vi "ZSlice compute-core.vi"(6 "ZStage Pos":dbl, 7 "Objective Pos Locked":bool, 8 "error in (no error)":errorcluster, 9 "ZStep":dbl, 10 "ZStop":dbl, 11 "ZStart":dbl) -> (0 "error out":errorcluster, 1 "Motor Z Planes(um)":dbl[](array[numeric]) format="%#_12f", 2 "# of Z-planes":i32, 3 "AOL Z Planes(um)":dbl[](array[numeric]) format="%#_12f", 5 "ZStagePos":dbl)   [LabVIEW 2020]
uses:
  <vilib>/imath/engines/lvmath2/RunTimeEngine/Managers/WorkSpace/UID Generator.vi
  <vilib>/imath/engines/lvmath2/RunTimeEngine/BuiltInFunctions/abs/NIMS_abs(signed).vi
  <instcachedir>/0/NIMS_abs(signed)_C4FCB8E6058B49B797C7C8D53CA5F6EC.lvgen/NIMS_abs(signed)_C4FCB8E6058B49B797C7C8D53CA5F6EC_000.vi
  <vilib>/imath/engines/lvmath2/RunTimeEngine/BuiltInFunctions/round/NIMS_round(DBL-S).vi
  <vilib>/imath/engines/lvmath2/RunTimeEngine/BuiltInFunctions/zeros/NIMS_V=zeros(I32,I32).vi
  <vilib>/imath/engines/lvmath2/RunTimeEngine/RunTimeType/NIMS_RunTimeType_From StrictType (excl LVString).vi
  <instcachedir>/0/NIMS_RunTimeType_From StrictType (excl LVString)_867E31CEF7BF4ABF8B0CFC3D01EB2647.lvgen/NIMS_RunTimeType_From StrictType (excl LVString)_867E31CEF7BF4ABF8B0CFC3D01EB2647_000.vi
  <vilib>/imathl/engines/lvmath/Functions/Error Handling/Create Error.vi
  <vilib>/imath/engines/lvmath2/RunTimeEngine/LocalVariableDefStatement/MC_LocalVariableDefStatement_Display.vi
  <vilib>/imath/engines/lvmath2/RunTimeEngine/RangeToken/NIMS_Range_R2 - Float.vi
  <instcachedir>/0/NIMS_Range_R2 - Float_1157773CA8584B2296CF3B05309B9E35.lvgen/NIMS_Range_R2 - Float_1157773CA8584B2296CF3B05309B9E35_000.vi
  <vilib>/imath/engines/lvmath2/RunTimeEngine/CommandStatement/MC_CommandStatement_break.vi
  <vilib>/imath/engines/lvmath2/RunTimeSupport/NIMS_Error if Not Equal.vi
  <instcachedir>/0/NIMS_Error if Not Equal_7DE3326BD2F940169CB4472B06005DF0.lvgen/NIMS_Error if Not Equal_7DE3326BD2F940169CB4472B06005DF0_000.vi
  <vilib>/imath/engines/lvmath2/RunTimeEngine/IndexReplace/NIMS M(S,S)=S.vi
  <instcachedir>/0/NIMS M(S,S)=S_399908DFD004401BA66ACC94B4F53E50.lvgen/NIMS M(S,S)=S_399908DFD004401BA66ACC94B4F53E50_000.vi
  <vilib>/imath/engines/lvmath2/RunTimeEngine/ErrorHandling/NIMS_Create Error From Enums.vi
  <vilib>/imath/engines/lvmath2/RunTimeEngine/NodeEndStatement/NIMS_NodeEndStatement_Get Vector.vi
  <instcachedir>/0/NIMS_NodeEndStatement_Get Vector_A95D2DB2A9BC46BA8CD6C6E4D7235685.lvgen/NIMS_NodeEndStatement_Get Vector_A95D2DB2A9BC46BA8CD6C6E4D7235685_001.vi
  <vilib>/imath/engines/lvmath/Functions/Error Handling/MergeErrorsWrapper.vi
  <vilib>/imath/engines/lvmath2/RunTimeEngine/Managers/SymbolTable/Clear UID.vi
  <vilib>/imath/engines/lvmath2/RunTimeEngine/NodeEndStatement/NIMS_NodeEndStatement_Output.vi
  <instcachedir>/0/NIMS_NodeEndStatement_Output_53EC0D466D134D7ABD903AC30B43404B.lvgen/NIMS_NodeEndStatement_Output_53EC0D466D134D7ABD903AC30B43404B_005.vi
  <instcachedir>/0/NIMS_NodeEndStatement_Output_53EC0D466D134D7ABD903AC30B43404B.lvgen/NIMS_NodeEndStatement_Output_53EC0D466D134D7ABD903AC30B43404B_001.vi
  <vilib>/imath/engines/lvmath2/RunTimeEngine/ErrorHandling/NIMS_Finalize Error.vi
  <vilib>/imath/engines/lvmath2/RunTimeEngine/Managers/SymbolTable/NIMS_WorkSpace.lvlib
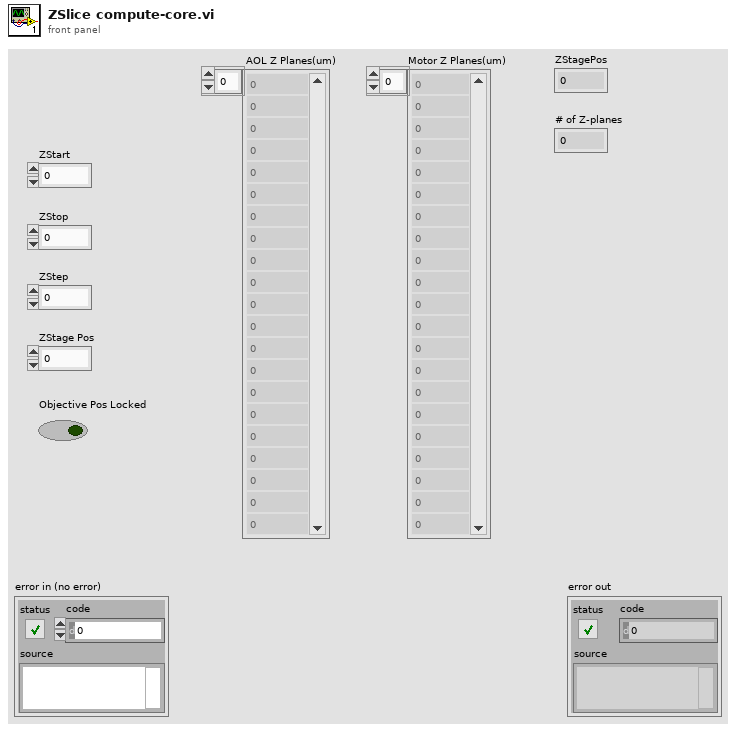
[diagram p1: front panel]
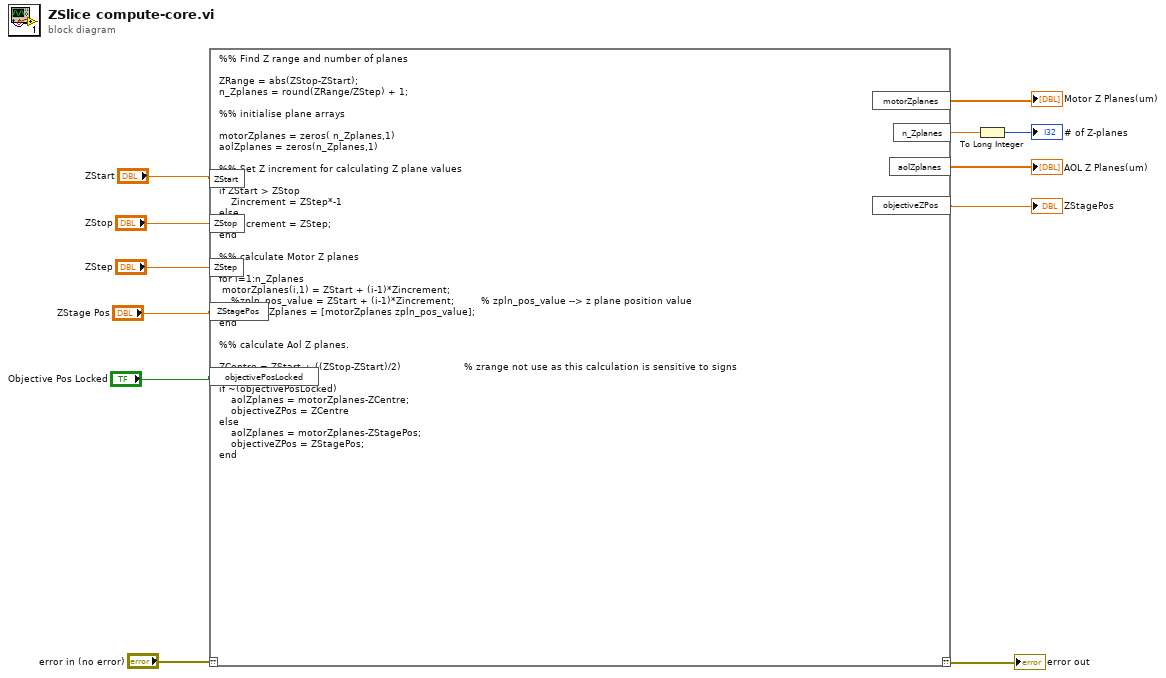
[diagram p0: block diagram]
diagram:
  n1 = mathscript code="%% Find Z range and number of planes\n\nZRange = abs(ZStop-ZStart);\nn_Zplanes = round(ZRange/ZStep) + 1;\n\n%% initialise plane arrays \n\nmotorZplanes = zeros( n_Zplanes,1)\naolZplanes = zeros(n_Zplanes,1)\n\n%% Set Z increment for calculating Z plane values\n\nif ZStart > ZStop\n    Zincrement = ZStep*-1\nelse\n    Zincrement = ZStep;\nend\n\n%% calculate Motor Z planes\n\nfor i=1:n_Zplanes\n motorZplanes(i,1) = ZStart + (i-1)*Zincrement;\n    %zpln_pos_value = ZStart + (i-1)*Zincrement;         % zpln_pos_value --> z plane position value\n    %motorZplanes = [motorZplanes zpln_pos_value];\nend\n\n%% calculate Aol Z planes.\n\nZCentre = ZStart + ((ZStop-ZStart)/2)                     % zrange not use as this calculation is sensitive to signs\n\nif ~(objectivePosLocked)\n    aolZplanes = motorZplanes-ZCentre;\n    objectiveZPos = ZCentre\nelse\n    aolZplanes = motorZplanes-ZStagePos;\n    objectiveZPos = ZStagePos;      \nend"("??"="error in (no error)", "ZStart"="ZStart", "ZStop"="ZStop", "ZStep"="ZStep", "ZStagePos"="ZStage Pos", "objectivePosLocked"="Objective Pos Locked") -> ("??"=→"error out":errorcluster, "n_Zplanes"=w7:dbl, "motorZplanes"=→"Motor Z Planes(um)":dbl[], "aolZplanes"=→"AOL Z Planes(um)":dbl[], "objectiveZPos"=→"ZStagePos":dbl)
  n2 = To Long Integer(number=w7) -> (32bit integer=→"# of Z-planes":i32)
